vi "Version Scripting.vi"(9 "Project":refnum<vi>, 10 "To":T1, 11 "From":T1) -> ()   [LabVIEW 2020]
uses:
  Version.ctl
  Tags.ctl
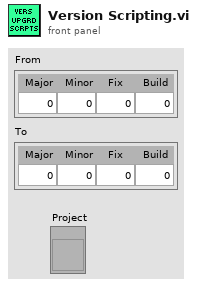
[diagram p1: front panel]
types:
  T1 = typedef "Version.ctl" = cluster{"Major":u16, "Minor":u16, "Fix":u16, "Build":u16}
  T2 = typedef "Tags.ctl" = enum16{"sol.reversi.version"}
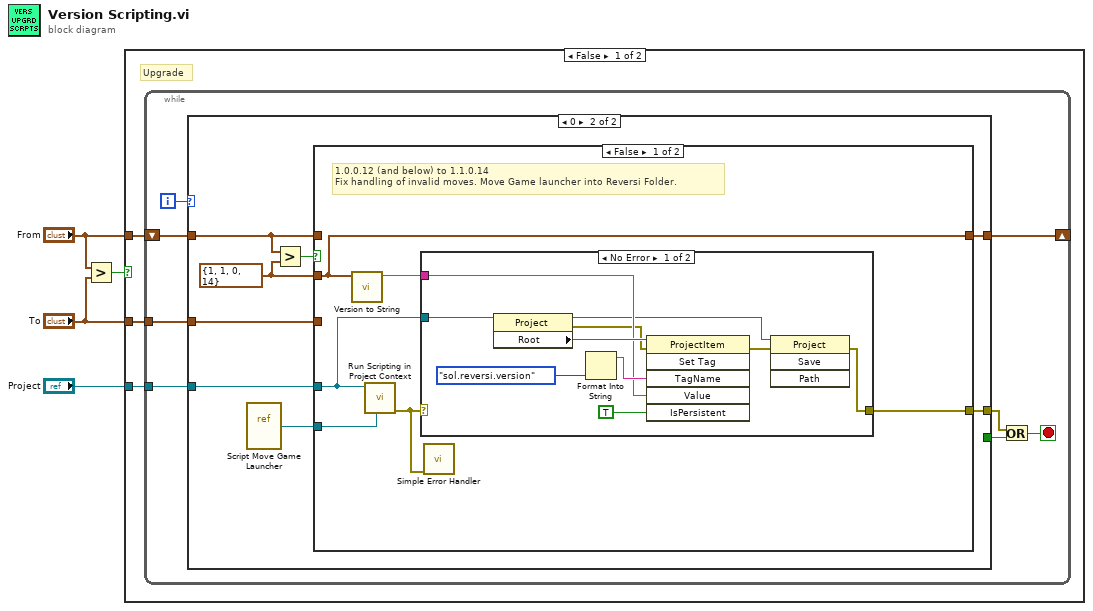
[diagram p0: block diagram]
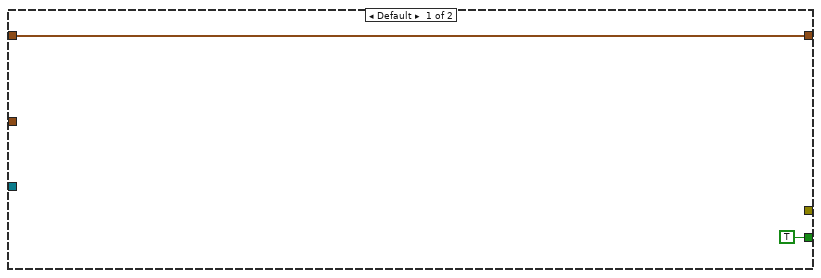
[diagram p2: hidden frame]
diagram:
  n1 = Greater?(x="From", y="To") -> (0:w1:bool)
  n2 = case shown="False" w1 {
    tunnel: "Project" -> [w7 _]
    tunnel: "From" -> [w6 _]
    tunnel: "To" -> [w5 _]
    frame False {
      # "Upgrade"
      n3 = while {
        shift-right: [w13] -> _
        shift-left: w6 -> [w14]
        tunnel: w7 -> [w10]
        tunnel: w5 -> [w12]
        i -> [w15]
        stop <- w9 stop-if-true
        n4 = case shown="0" w15 {
          tunnel: w14 -> [w16 w23]
          tunnel: [w16 w22] -> w13
          tunnel: w12 -> [_ w21]
          tunnel: [TRUE _] -> w11
          tunnel: w10 -> [_ w20]
          tunnel: [_ w19] -> w8
          frame Default {
          }
          frame 0 {
            w24 = T1 {"Major"=1, "Minor"=1, "Fix"=0, "Build"=14} ("y")
            n5 = vi-ref "Script Move Game Launcher.vi"() -> (w18:refnum<vi>)
            n6 = Greater?(x=w23, y=w24) -> (0:w25:bool)
            n7 = case shown="False" w25 {
              tunnel: w24 -> [w31 _]
              tunnel: w23 -> [_ w43]
              tunnel: [w31 w43] -> w22
              tunnel: w21 -> [_ _]
              tunnel: w20 -> [w28 _]
              tunnel: [w30 _] -> w19
              tunnel: w18 -> [w27 _]
              frame False {
                # "1.0.0.12 (and below) to 1.1.0.14\nFix handling of invalid moves. Move Game launcher into Reversi Folder."
                n8 = call "Version to String.vi"("Version"=w31) -> ("Version String"=w29:string)  [unwired: 10 in]
                n9 = call "Run Scripting in Project Context.vi"("Scripting VI"=w27, "Project"=w28) -> ("error out"=w26:errorcluster)  [unwired: 9 in]
                n10 = case shown="No Error" w26 {
                  selector: w26 -> [_ w42]
                  tunnel: [w41 w42] -> w30
                  tunnel: w29 -> [w37 _]
                  tunnel: w28 -> [w32 _]
                  frame No Error {
                    n11 = property class="Project"(reference=w32) -> (reference out=w34:refnum<vi>, error out=w35:errorcluster, "Root"=w40:refnum<vi>)  [unwired: 1 in]
                    n12 = Format Into String(Tags."sol.reversi.version" ("Tags")) -> (resulting string=w38:string)  [unwired: 3 in, 1 out]
                    n13 = invoke class="ProjectItem" method="Set Tag"(reference=w40, error in=w35, "TagName"=w38, "Value"=w37, "IsPersistent"=TRUE ("Is Persistent (T)")) -> (error out=w33:errorcluster)  [unwired: 1 in, 5 out]
                    n14 = invoke class="Project" method="Save"(reference=w34, error in=w33) -> (error out=w41:errorcluster)  [unwired: 2 in, 3 out]
                  }
                  frame Error {
                  }
                }
                n15 = call <vilib>:"Simple Error Handler.vi"("error in (no error)"=w26) -> ()  [unwired: 4 in, 5 out]
              }
              frame True {
                # "Already greater than 1.0.0.21, nothing to do for this step."
              }
            }
          }
        }
        n16 = Or(x=w8, y=w11) -> (x .or. y?=w9:bool)
      }
    }
    frame True {
      # "Downgrade"
    }
  }
